vi "Verify Core.vi"(8 "error in":errorcluster, 10 "Test Data":string) -> (0 "error out":errorcluster, 1 "Failure Message":string, 2 "Passed?":bool)   [LabVIEW 2020, in "Approval Tests.lvlib"]
doc: "Performs an approval test.\n\nThe first call, the test passes and the test data is written to the approved file.\n\nOn subsequent runs the test data is compared to the contents of the approved file.\nIf it is a match, the test passes.\nIf it is not a match, the test fails and the test data is written to the actual file.\n\nAt the point the user can diff the approved and actual files and determine if they approve of the changes or not. If they approve, they replace the old approved file with the actual file. \n\nNOTE: You should keep the approved files in Source Code Control. You should ignore *.actual in your .gitignore file - there is no need to store those."
uses:
  Approval Tests.lvlib
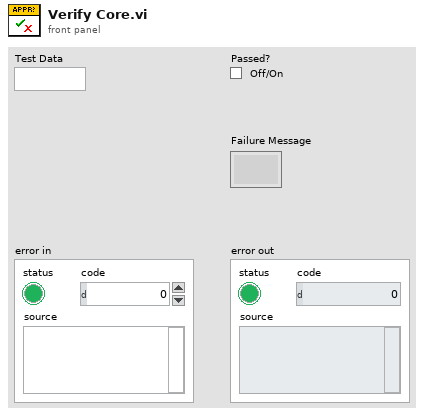
[diagram p1: front panel]
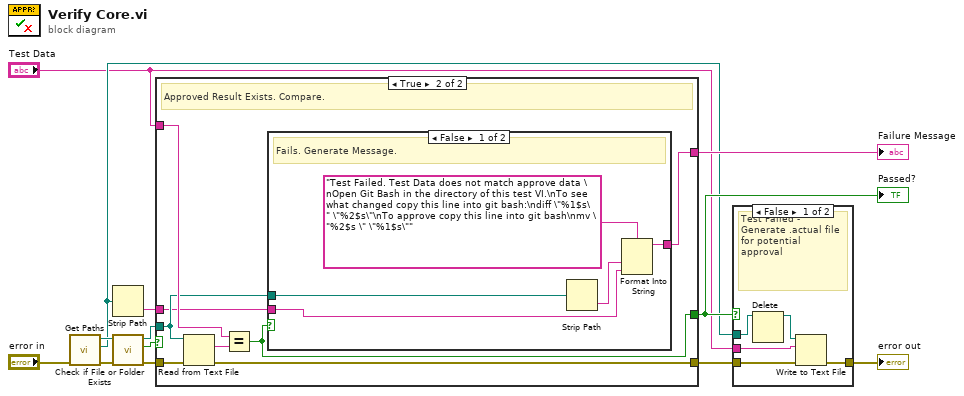
[diagram p0: block diagram]
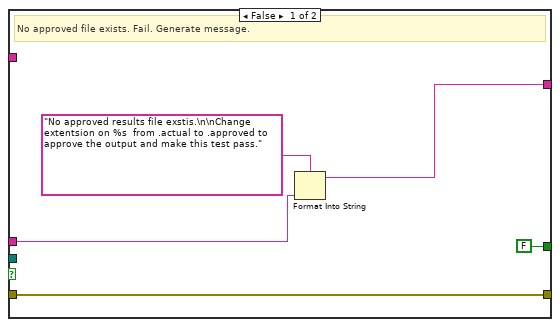
[diagram p3: hidden frame]
diagram:
  n1 = call "Get Paths.vi"("error in"="error in") -> ("error out"=w12:errorcluster, "actual path"=w3:path, "approved path"=w5:path)  [unwired: 8 in]
  n2 = Strip Path(path=w3) -> (name=w2:string)  [unwired: 1 out]
  n3 = call <vilib>:"Check if File or Folder Exists.vi"("error in (no error)"=w12, "path"=w5) -> ("error out"=w11:errorcluster, "file or folder exists?"=w7:bool, "dup path"=w8:path)  [unwired: 7 in]
  n4 = case shown="True" w7 {
    tunnel: "Test Data" -> [_ w22]
    tunnel: [w18 w25] -> w10
    tunnel: w11 -> [w18 w26]
    tunnel: w8 -> [_ w20]
    tunnel: [FALSE ("Passed?") w23] -> w4
    tunnel: [w14 w21] -> w6
    tunnel: w2 -> [w16 w19]
    frame False {
      # "No approved file exists. Fail. Generate message."
      n5 = Format Into String(format string="No approved results file exstis.\n\nChange extentsion on %s  from .actual to .approved to approve the output and make this test pass.", w16) -> (resulting string=w14:string)  [unwired: 2 in, 1 out]
    }
    frame True {
      # "Approved Result Exists. Compare."
      n6 = Read from Text File(file (use dialog)=w20, error in=w26) -> (text=w24:string, error out=w25:errorcluster)  [unwired: 2 in, 2 out]
      n7 = Equal?(x=w22, y=w24) -> (x = y?=w23:bool)
      n8 = case shown="False" w23 {
        tunnel: [w31 _] -> w21
        tunnel: w20 -> [w28 _]
        tunnel: w19 -> [w27 _]
        frame False {
          # "Fails. Generate Message."
          n9 = Strip Path(path=w28) -> (name=w29:string)  [unwired: 1 out]
          n10 = Format Into String(format string="Test Failed. Test Data does not match approve data \nOpen Git Bash in the directory of this test VI.\nTo see what changed copy this line into git bash:\ndiff \"%1$s\" \"%2$s\"\nTo approve copy this line into git bash\nmv \"%2$s \" \"%1$s\"", w29, w27) -> (resulting string=w31:string)  [unwired: 2 in, 1 out]
        }
        frame True {
          # "Passes. No Message Needed.."
        }
      }
    }
  }
  "Passed?" <- w4
  "Failure Message" <- w6
  n11 = case shown="False" w4 {
    tunnel: w10 -> [w35 w37]
    tunnel: [w36 w37] -> w9
    tunnel: w3 -> [w34 _]
    tunnel: "Test Data" -> [w32 _]
    frame False {
      # "Test Failed - Generate .actual file for potential approval"
      n12 = Delete(path (use dialog)=w34) -> (deleted path=w33:path)  [unwired: 4 in, 2 out]
      n13 = Write to Text File(file (use dialog)=w33, text=w32, error in=w35) -> (error out=w36:errorcluster)  [unwired: 1 in, 2 out]
    }
    frame True {
      # "Passed - no need for .actual file"
    }
  }
  "error out" <- w9
